vi "Read hours.vi"(8 "error in (no error)":errorcluster, 11 "ClockTimes in":refnum<class "ClockTimes.lvclass">) -> (0 "error out":errorcluster, 2 "hours":dbl[unit] min=0.0 max=86400.0, 3 "ClockTimes out":refnum<class "ClockTimes.lvclass">)   [LabVIEW 2022 SP3, in "TCSDataDefinitions.lvlib" / "TCSPublicStatus.lvlib" / "CurrentTimes.lvlib" / "ClockTimes.lvclass"]
uses:
  ClockTimes.lvclass
  ClockTimes.lvclass/ClockTimes.ctl
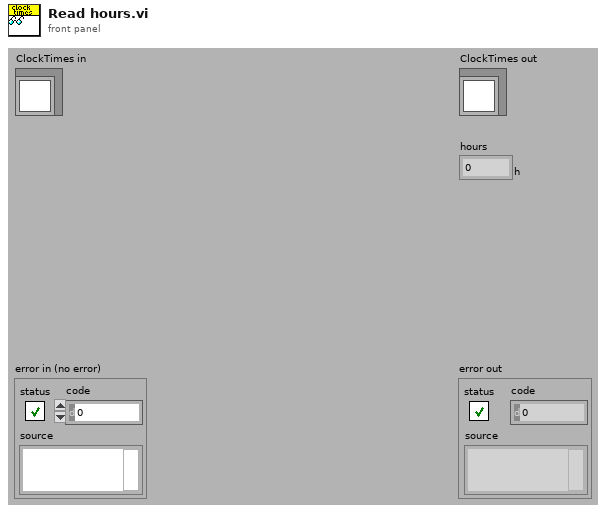
[diagram p1: front panel]
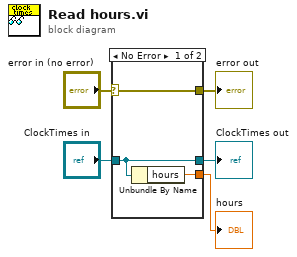
[diagram p0: block diagram]
diagram:
  n1 = case shown="No Error" "error in (no error)" {
    selector: "error in (no error)" -> [w8 w9]
    tunnel: [w8 w9] -> w4
    tunnel: [w7 w10] -> w2
    tunnel: "ClockTimes in" -> [w7 w10]
    tunnel: [w6 _] -> w1
    frame No Error {
      n2 = Unbundle By Name(w7) -> ("hours"=w6:dbl[unit])
    }
    frame Error {
    }
  }
  "error out" <- w4
  "ClockTimes out" <- w2
  "hours" <- w1
